vi "Extract Single Tone Information N Chan.vi"(6 "advanced search":T4={"approx freq. (optional)"=-1.0, "search (+/- % of Fsampl.)"=5.0} {"search (+/- % of Fsampl.)" format="%0.2p"; "approx freq. (optional)" format="%0.2p"}, 8 "error in (no error)":errorcluster, 10 "export mode":T3(ring), 11 "time signals in":waveform(dbl)[](array[waveform])) -> (0 "error out":errorcluster, 1 "detected phases (deg)":dbl[](array[numeric]) format="%.2p", 2 "detected amplitudes":dbl[](array[numeric]) format="%.2p", 3 "detected frequencies":dbl[](array[numeric]) format="%.2p", 4 "measurements info":T2(array[cluster]) {"uncertainty" format="%0.2p"}, 5 "exported signals":T1(array[cluster]) {"exported spectrum (dB)"."dB Spectrum (Hann)" format="%.2p"; "exported spectrum (dB)"."df" format="%.2p"; "exported spectrum (dB)"."f0" format="%.2p"})   [LabVIEW 2020, in "NI_MAPro.lvlib"]
doc: "Takes a signal in, finds the single tone with the highest amplitude or searches a specified frequency range, and returns the single tone frequency, amplitude, and phase. The input signal can be real or complex and single-channel or multichannel. Wire data to the <B>time signal in</B> input to determine the polymorphic instance to use or manually select the instance."
uses:
  NI_MAPro.lvlib
  NI_MABase.lvlib
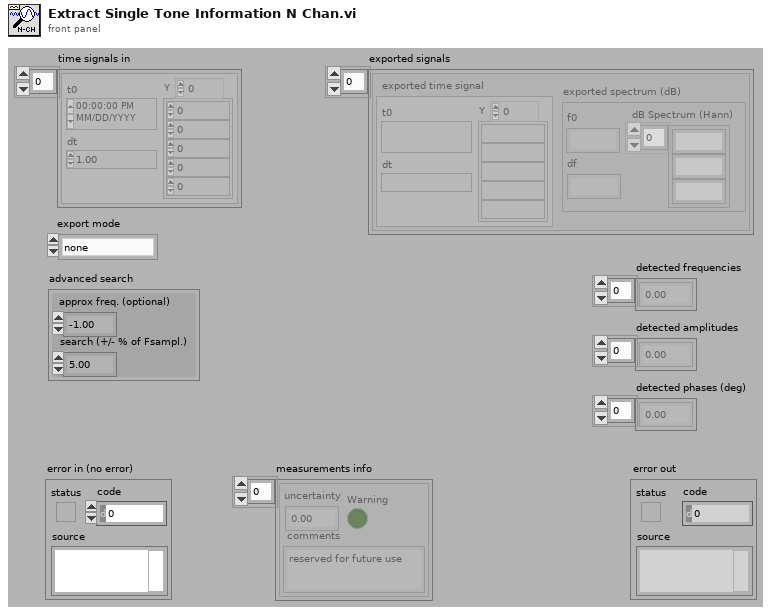
[diagram p1: front panel]
types:
  T1 = cluster{"exported time signal":waveform(dbl), "exported spectrum (dB)":cluster{"f0":dbl, "df":dbl, "dB Spectrum (Hann)":dbl[]}}[]
  T2 = cluster{"uncertainty":dbl, "Warning":bool, "comments":string}[]
  T3 = enum32{"none", "input signal", "detected signal", "residual signal"}
  T4 = cluster{"approx freq. (optional)":dbl, "search (+/- % of Fsampl.)":dbl}
  T5 = cluster{"uncertainty":dbl, "Warning":bool, "comments":string}
  T6 = cluster{"exported time signal":waveform(dbl), "exported spectrum (dB)":cluster{"f0":dbl, "df":dbl, "dB Spectrum (Hann)":dbl[]}}
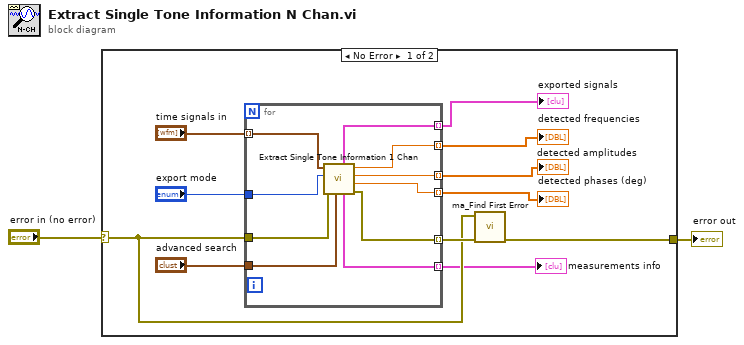
[diagram p0: block diagram]
diagram:
  n1 = case shown="No Error" "error in (no error)" {
    selector: "error in (no error)" -> [w4 w24]
    tunnel: [w5 w24] -> w1
    frame No Error {
      n2 = for {
        tunnel: "advanced search" -> [w19]
        tunnel: [w17] -> w12 mode=indexing
        tunnel: [w16] -> w11 mode=indexing
        tunnel: [w15] -> w10 mode=indexing
        tunnel: "export mode" -> [w22]
        tunnel: "time signals in" -> [w23] mode=indexing
        tunnel: [w18] -> w7 mode=indexing
        tunnel: w4 -> [w21]
        tunnel: [w20] -> w6 mode=indexing
        tunnel: [w14] -> w3 mode=indexing
        n3 = call "Extract Single Tone Information 1 Chan.vi"("advanced search"=w19, "error in (no error)"=w21, "export mode"=w22, "time signal in"=w23) -> ("error out"=w20:errorcluster, "detected phase (deg)"=w15:dbl, "detected amplitude"=w16:dbl, "detected frequency"=w17:dbl, "measurement info"=w14:T5, "exported signals"=w18:T6)  [unwired: 2 out]
      }
      "detected phases (deg)" <- w10
      "detected frequencies" <- w12
      "detected amplitudes" <- w11
      "measurements info" <- w3
      "exported signals" <- w7
      n4 = call "ma_Find First Error.vi"("error array in"=w6, "error in 1 (no error)"=w4) -> ("error out"=w5:errorcluster)  [unwired: 2 in, 3 out]
    }
    frame Error {
    }
  }
  "error out" <- w1
